vi "Wait For Read Buffer.vi"(8 "error in (no error)":errorcluster, 9 "BufferSize":i32, 10 "timeout (ms)":i32=5000, 11 "AI Tasks":T1[](array[typedef])) -> (0 "error out":errorcluster={"status"=FALSE, "code"=555, "source"="Timed out waiting for Signal Bank."})   [LabVIEW 2020]
uses:
  Type Defs/Task Struct.ctl
  <resource>/objmgr/daqmx.rc
panel:
  out "NumAvail":u32
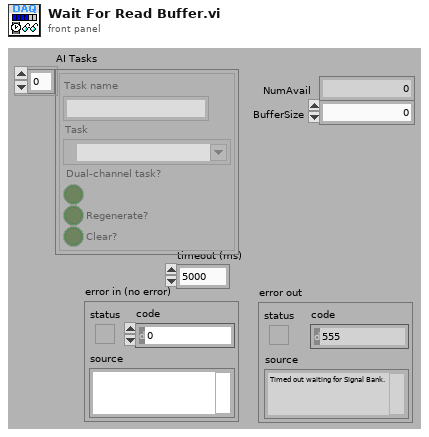
[diagram p1: front panel]
types:
  T1 = typedef "Task Struct.ctl" = cluster{"Task name":string, "Task":refnum<k21>, "Dual-channel task?":bool, "Regenerate?":bool, "Clear?":bool}
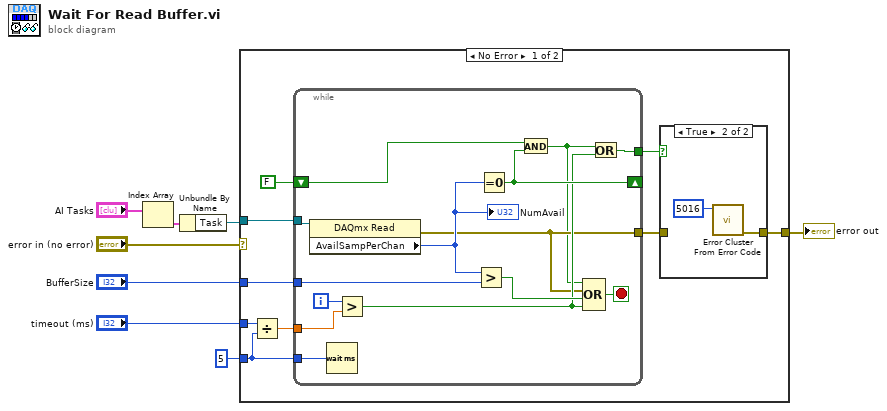
[diagram p0: block diagram]
diagram:
  n1 = Index Array(array="AI Tasks") -> (element=w6:T1)  [unwired: 1 in]
  n2 = Unbundle By Name(w6) -> ("Task"=w5:refnum<k21>)
  n3 = case shown="No Error" "error in (no error)" {
    selector: "error in (no error)" -> [_ w35]
    tunnel: "timeout (ms)" -> [w17 _]
    tunnel: w5 -> [w15 _]
    tunnel: "BufferSize" -> [w13 _]
    tunnel: [w16 w35] -> w2
    tunnel: 5 -> [w9 _]
    frame No Error {
      n4 = Divide(x=w17, y=w9) -> (x/y=w10:dbl)
      n5 = while {
        tunnel: w10 -> [w23]
        tunnel: w15 -> [w30]
        tunnel: [w22] -> w14
        tunnel: w13 -> [w31]
        shift-right: [w28] -> _
        shift-left: FALSE -> [w27]
        tunnel: [w26] -> w11
        tunnel: w9 -> [w24]
        i -> [w33]
        stop <- w34 stop-if-true
        n6 = property class="DAQmx Read"(reference=w30) -> (error out=w22:errorcluster, "AvailSampPerChan"=w29:u32)  [unwired: 1 in, 1 out]
        "NumAvail" <- w29
        n7 = Wait (ms)(milliseconds to wait=w24) -> ()  [unwired: 1 out]
        n8 = Greater?(x=w33, y=w23) -> (0:w25:bool)
        n9 = Greater?(x=w29, y=w31) -> (0:w32:bool)
        n10 = Equal To 0?(x=w29) -> (x = 0?=w28:bool)
        n11 = And(x=w27, y=w28) -> (x .and. y?=w21:bool)
        n12 = Compound Arithmetic op=OR(w21, w22, w32, w25) -> (w34:bool)
        n13 = Or(x=w21, y=w25) -> (x .or. y?=w26:bool)
      }
      n14 = case shown="True" w11 {
        tunnel: [w18 w20] -> w16
        tunnel: w14 -> [w18 _]
        frame False {
        }
        frame True {
          n15 = call <vilib>:"Error Cluster From Error Code.vi"("error code (0)"=5016) -> ("error out"=w20:errorcluster)  [unwired: 8 in]
        }
      }
    }
    frame Error {
    }
  }
  "error out" <- w2
